vi "stageFindCell_v5.vi"(0 "stage in":T5={"Actuator COM"="COM14", "Actuator type"=enum."Scientifica"}, 1 "slice image":T3, 5 "cell index":i32, 7 "transform cluster + actuator":T1, 9 "cell match score":sgl=500.0, 11 "error in":errorcluster, 12 "cell images":T3[](array[typedef])) -> (3 "found":T3(plugin-control), 4 "stageout":T5={"Actuator COM"="COM14", "Actuator type"=enum."Scientifica"}, 6 "cell found":bool, 10 "screen cell location (px)":i32[](array[numeric]), 14 "Score":sgl, 15 "error out":errorcluster)   [LabVIEW 2015]
uses:
  <vilib>/vision/NI_Vision_Development_Module.lvlib
  pipette cleaning/pressure box/cleaning_soft/controls/actuator_type.ctl
  pipette cleaning/pressure box/cleaning_soft/controls/actuator_cluster.ctl
  <vilib>/vision/Image Controls.llb/IMAQ Image.ctl
  machine_vision/coordinate model vis/transform_properties_actuators.ctl
  machine_vision/controls/transform_cluster_actuator.ctl
panel:
  out "Y Resolution":i32
  out "X Resolution":i32
  in  "z moves":i32[](array[numeric])=[0, 10, 10, 10, 10, 10, 10, 10, 10, 10, 10, 10, 10, 10, 10, 10, -150, -10, -10, -10, -10, -10, -10, -10, -10, -10, -10, -10, -10, -10, -10, -10, 150]
  in  "Algorithm":i32(ring)=1 items=["All", "Low Discrepancy Sampling", "Grayscale Value Pyramid", "Gradients Pyramid"]
  out "Number of Matches Found":i32
  out "Matches (pixel)":T2(array[cluster]) {"Bounding Box"."y" format="%.2f"; "Bounding Box"."x" format="%.2f"; "Score" format="%.2f"; "Scale" format="%.2f"; "Angle" format="%.2f"; "Position"."y" format="%.2f"; "Position"."x" format="%.2f"}
  in  "autofocus on?":bool=TRUE
  in  "Match Parameters":T4={"Number of Matches Requested"=1, "Minimum Match Score"=500.0, "Angle Ranges"=[]} {"Angle Ranges"."End Angle" min=-360 max=360; "Angle Ranges"."Start Angle" min=-360 max=360; "Minimum Match Score" min=0 max=1000; "Number of Matches Requested" min=1 max=9999}
  # "last element brings it to 0"
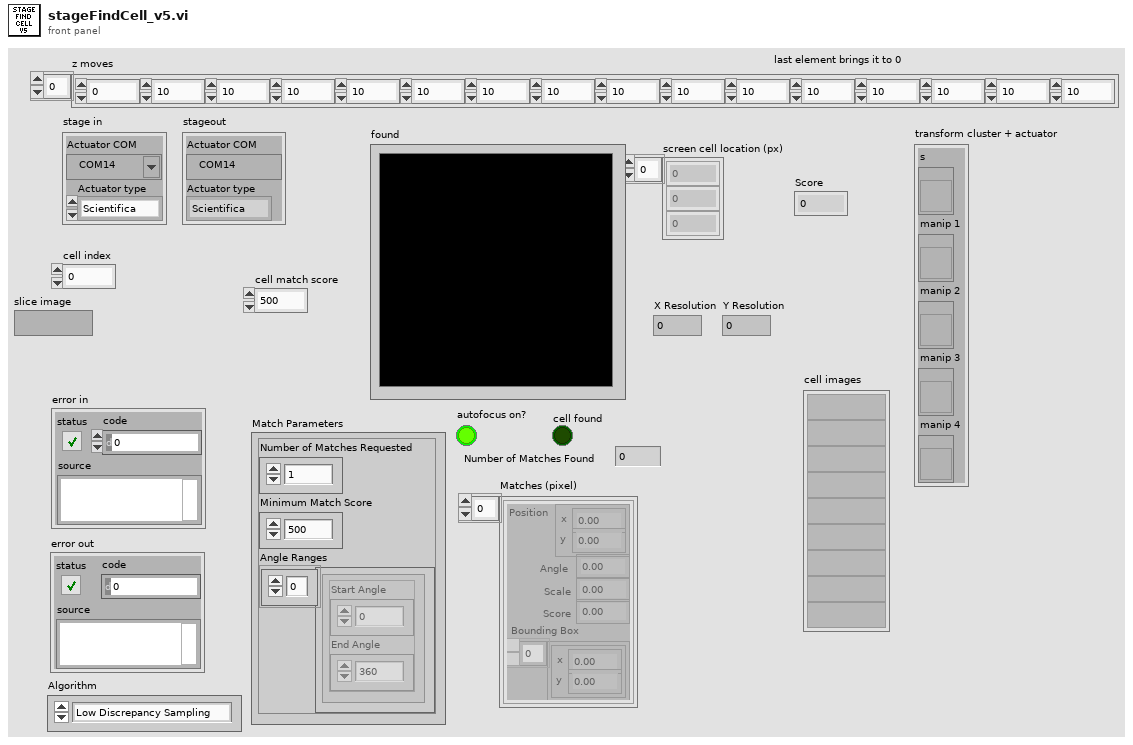
[diagram p1: front panel]
types:
  T1 = typedef "transform_cluster_actuator.ctl" = cluster{"s":refnum<vi>, "manip 1":refnum<vi>, "manip 2":refnum<vi>, "manip 3":refnum<vi>, "manip 4":refnum<vi>}
  T2 = cluster{"Position":cluster{"x":sgl, "y":sgl}, "Angle":sgl, "Scale":sgl, "Score":sgl, "Bounding Box":cluster{"x":sgl, "y":sgl}[]}[]
  T3 = typedef "IMAQ Image.ctl" = refnum<image>
  T4 = cluster{"Number of Matches Requested":i32, "Minimum Match Score":sgl, "Angle Ranges":cluster{"Start Angle":sgl, "End Angle":sgl}[]}
  T5 = typedef "actuator_cluster.ctl" = cluster{"Actuator COM":refnum<visa-resource-name>, "Actuator type":T6}
  T6 = typedef "actuator_type.ctl" = enum16{"Scientifica", "Sutter", "Demo", "Off"}
  T7 = typedef "Image Type" = u32
  T8 = cluster{"Position":cluster{"x":sgl, "y":sgl}, "Angle":sgl, "Scale":sgl, "Score":sgl, "Bounding Box":cluster{"x":sgl, "y":sgl}[]}
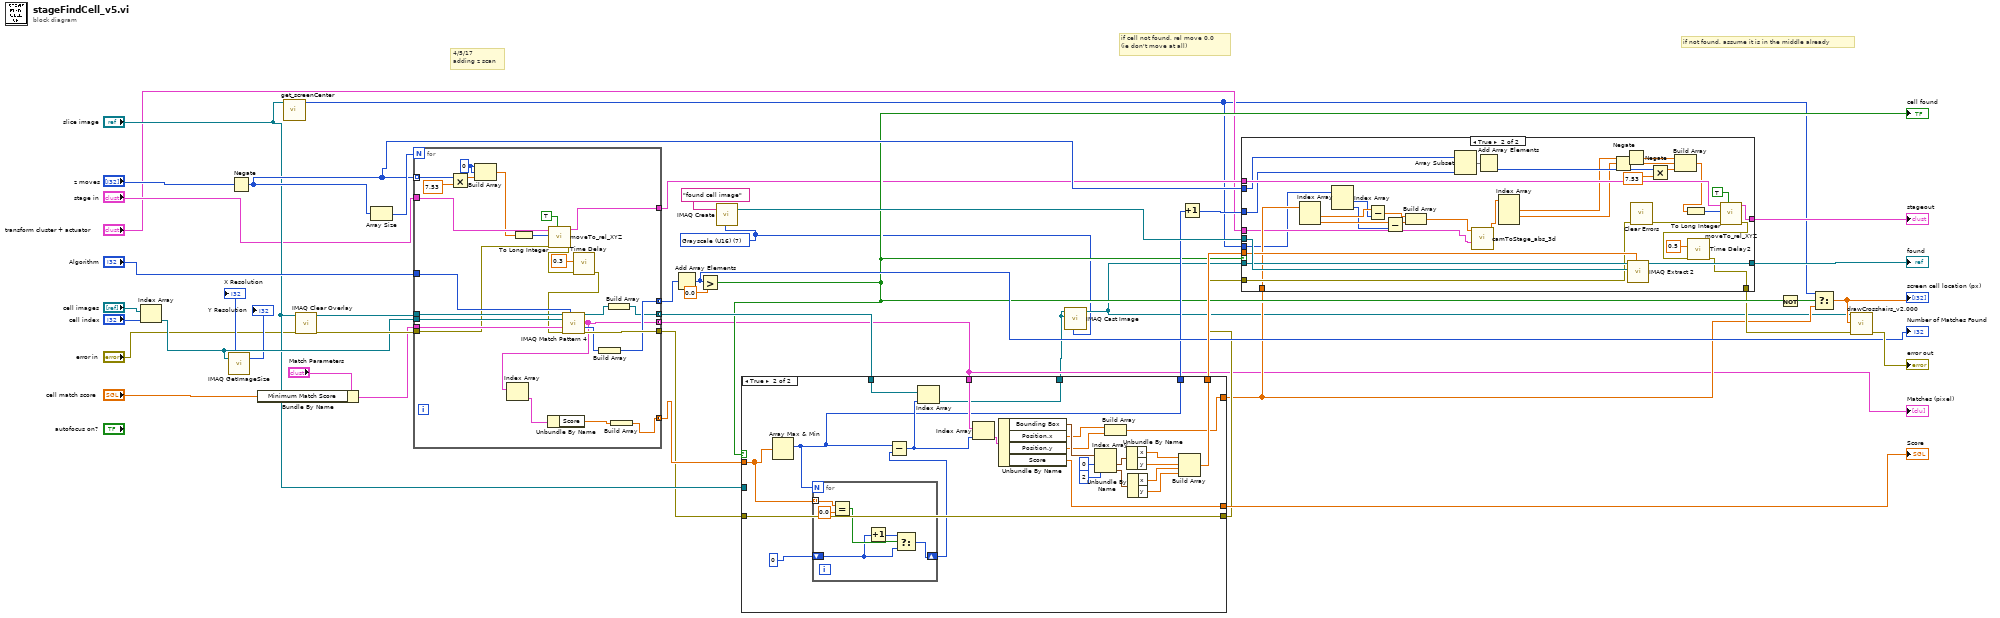
[diagram p0: block diagram]
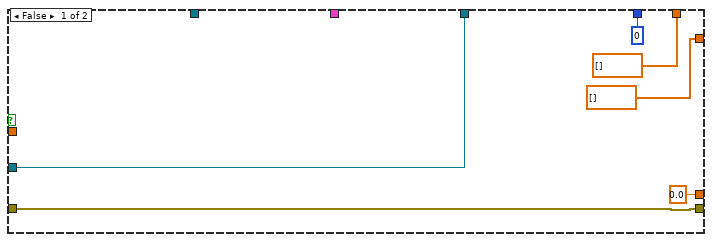
[diagram p2: hidden frame]
diagram:
  w1 = T7 7 items=["Grayscale (U8)", "Grayscale (I16)", "Grayscale (SGL)", "Complex (CSG)", "RGB (U32)", "HSL (U32)", "RGB (U64)", "Grayscale (U16)"] ("Image Type")
  # "if not found, assume it is in the middle already"
  # "4/5/17\nadding z scan"
  # "if cell not found, rel move 0,0\n(ie don't move at all)"
  n1 = Index Array(array="cell images", index="cell index") -> (element=w31:T3)
  n2 = call "IMAQ GetImageSize"("Image"=w31) -> ("Y Resolution"=→"Y Resolution":i32, "X Resolution"=→"X Resolution":i32)  [unwired: 3 in, 1 out]
  n3 = Negate(x="z moves") -> (-x=w20:i32[])
  n4 = Bundle By Name(cluster="Match Parameters", "Minimum Match Score"="cell match score") -> (w37:T4)
  n5 = call "get_screenCenter.vi"("image"="slice image") -> ("screen center (px)"=w5:i32[])  [unwired: 10 in]
  n6 = call "IMAQ Clear Overlay"("error in (no error)"="error in", "Image"="slice image") -> ("error out"=w43:errorcluster, "Image Out"=w34:T3)  [unwired: 8 in]
  n7 = Array Size(array=w20) -> (size(s)=w26:i32)
  n8 = for {
    N: w26 -> [_]
    tunnel: w31 -> [w70]
    tunnel: [w50] -> w4 mode=concatenating
    tunnel: w37 -> [w69]
    tunnel: w34 -> [w71]
    tunnel: [w47] -> w21 mode=concatenating
    tunnel: w43 -> [w55]
    tunnel: [w68] -> w14
    tunnel: "stage in" -> [w67]
    tunnel: w20 -> [w66] mode=indexing
    tunnel: [w63] -> w11
    tunnel: [w52] -> w24 mode=concatenating
    tunnel: "Algorithm" -> [w60]
    tunnel: [w49] -> w22 mode=concatenating
    w65 = 0 ("element")
    n9 = Multiply(x=w66, y=7.53) -> (x*y=w62:dbl)
    n10 = Build Array(w65, w65, w62) -> (w64:dbl[])
    n11 = To Long Integer(number=w64) -> (32bit integer=w56:i32[])
    n12 = call "moveTo_rel_XYZ.vi"("blocking?"=TRUE, "error in"=w55, "XYZ location (steps)"=w56, "Actuator cluster in"=w67) -> ("error out"=w57:errorcluster, "Actuator cluster out"=w63:T5)  [unwired: 6 in]
    n13 = call "Time Delay"("error in (no error)"=w57, "Delay Time (s)"=0.3) -> ("error out"=w54:errorcluster)  [unwired: 9 in]
    n14 = call "IMAQ Match Pattern 4"("Image"=w71, "Algorithm"=w60, "Template Image"=w70, "Parameters"=w69, "error in (no error)"=w54) -> ("Image (duplicate)"=w48:T3, "Matches (pixel)"=w50:T2, "Number of Matches"=w53:i32, "error out"=w68:errorcluster)  [unwired: 6 in, 1 out]
    n15 = Index Array(array=w50) -> (element=w51:T8)  [unwired: 1 in]
    n16 = Unbundle By Name(w51) -> ("Score"=w46:sgl)
    n17 = Build Array(w53) -> (w52:i32[])
    n18 = Build Array(w48) -> (w47:T3[])
    n19 = Build Array(w46) -> (w49:sgl[])
  }
  "Matches (pixel)" <- w4
  n20 = Add Array Elements(numeric array=w24) -> (sum=w23:i32)
  "Number of Matches Found" <- w23
  n21 = Greater?(x=w23, y=0.0) -> (0:w16:bool)
  "cell found" <- w16
  n22 = call "IMAQ Create"("Image Name"="found cell image", "Image Type"=w1) -> ("New Image"=w40:T3)  [unwired: 3 in, 1 out]
  n23 = case shown="True" w16 {
    tunnel: [sgl[] [] w92] -> w41
    tunnel: [sgl[] [] w84] -> w6
    tunnel: [sgl 0.0 ("Score") w88] -> w28
    tunnel: w4 -> [_ w87]
    tunnel: w22 -> [_ w81]
    tunnel: w21 -> [_ w86]
    tunnel: [w76 w85] -> w3
    tunnel: [0 w78] -> w19
    tunnel: "slice image" -> [w76 _]
    tunnel: w14 -> [w72 w83]
    tunnel: [w72 w83] -> w13
    frame False {
    }
    frame True {
      n24 = Array Max & Min(array=w81) -> (max index (indices)=w78:i32)  [unwired: 3 out]
      n25 = for {
        N: w78 -> [_]
        tunnel: w81 -> [w107] mode=indexing
        shift-right: [w102] -> w79
        shift-left: 0 -> [w104]
        n26 = Equal?(x=w107, y=sgl 0.0) -> (x = y?=w105:bool)
        n27 = Increment(x=w104) -> (x+1=w103:i32)
        n28 = Select(t=w103, s=w105, f=w104) -> (s? t:f=w102:i32)
      }
      n29 = Subtract(x=w78, y=w79) -> (x-y=w82:i32)
      n30 = Index Array(array=w86, index=w82) -> (element=w85:T3)
      n31 = Index Array(array=w87, index=w82) -> (element=w101:T8)
      n32 = Unbundle By Name(w101) -> ("Bounding Box"=w91:cluster{"x":sgl, "y":sgl}[], "Position.x"=w90:sgl, "Position.y"=w89:sgl, "Score"=w88:sgl)
      n33 = Index Array(array=w91, index #1=0 ("index"), index #2=2 ("index")) -> (element #1=w98:cluster{"x":sgl, "y":sgl}, element #2=w97:cluster{"x":sgl, "y":sgl})
      n34 = Build Array(w90, w89) -> (w84:sgl[])
      n35 = Unbundle By Name(w98) -> ("x"=w94:sgl, "y"=w93:sgl)
      n36 = Unbundle By Name(w97) -> ("x"=w96:sgl, "y"=w95:sgl)
      n37 = Build Array(w94, w93, w96, w95) -> (w92:sgl[])
    }
  }
  "Score" <- w28
  n38 = call "IMAQ Cast Image"("Image Type"=w1, "Image Dst"=w3, "Image Src"=w3) -> ("Image Dst Out"=w2:T3)  [unwired: 7 in, 1 out]
  n39 = Increment(x=w19) -> (x+1=w18:i32)
  n40 = case shown="True" w16 {
    tunnel: w41 -> [_ w132]
    tunnel: w40 -> [w110 w145]
    tunnel: [w110 w144] -> w39
    tunnel: w2 -> [_ w143]
    tunnel: w11 -> [w108 w140]
    tunnel: w13 -> [w109 w129]
    tunnel: w20 -> [_ w136]
    tunnel: w18 -> [_ w135]
    tunnel: "transform cluster + actuator" -> [_ w121]
    tunnel: [w109 w126] -> w8
    tunnel: [w108 w125] -> w7
    tunnel: w6 -> [_ w123]
    tunnel: w5 -> [_ w120]
    frame False {
    }
    frame True {
      n41 = Index Array(array=w123) -> (element #1=w119:sgl, element #2=w117:sgl)  [unwired: 2 in]
      n42 = Index Array(array=w120) -> (element #1=w118:i32, element #2=w116:i32)  [unwired: 2 in]
      n43 = Subtract(x=w119, y=w118) -> (x-y=w115:sgl)
      n44 = Subtract(x=w117, y=w116) -> (x-y=w114:sgl)
      n45 = Build Array(w115, w114) -> (w113:sgl[])
      n46 = Array Subset(array=w136, length=w135) -> (w134:i32[])  [unwired: 1 in]
      n47 = call "camToStage_abs_3d.vi"("transform cluster + actuator"=w121, "abs pixel location"=w113) -> ("pipette location (steps)"=w122:dbl[])  [unwired: 9 in]
      n48 = Add Array Elements(numeric array=w134) -> (sum=w133:i32)
      n49 = Index Array(array=w122) -> (element #1=w131:dbl, element #2=w130:dbl)  [unwired: 3 in, 1 out]
      n50 = Negate(x=w130) -> (-x=w111:dbl)
      n51 = Negate(x=w131) -> (-x=w112:dbl)
      n52 = call "IMAQ Extract 2"("Optional Rectangle"=w132, "Image Dst"=w145, "Image Src"=w143) -> ("Image Dst Out"=w144:T3)  [unwired: 7 in, 1 out]
      n53 = call <vilib>:"Clear Errors.vi"("error in (no error)"=w129) -> ("error out"=w124:errorcluster)  [unwired: 5 in, 1 out]
      n54 = Multiply(x=w133, y=7.53) -> (x*y=w138:dbl)
      n55 = Build Array(w112, w111, w138) -> (w137:dbl[])
      n56 = To Long Integer(number=w137) -> (32bit integer=w142:i32[])
      n57 = call "moveTo_rel_XYZ.vi"("blocking?"=TRUE, "error in"=w124, "XYZ location (steps)"=w142, "Actuator cluster in"=w140) -> ("error out"=w127:errorcluster, "Actuator cluster out"=w125:T5)  [unwired: 6 in]
      n58 = call "Time Delay2"("error in (no error)"=w127, "Delay Time (s)"=0.5) -> ("error out"=w126:errorcluster)  [unwired: 9 in]
    }
  }
  "stageout" <- w7
  "found" <- w39
  n59 = Not(x=w16) -> (.not. x?=w35:bool)
  n60 = Select(t=w5, s=w35, f=w6) -> (s? t:f=w17:sgl[])
  "screen cell location (px)" <- w17
  n61 = call "drawCrosshairs_v2.000.vi"("error in (no error)"=w8, "pipette tip location (px)"=w17, "image in"=w2) -> ("error out"=→"error out":errorcluster)  [unwired: 7 in, 1 out]
